vi "REF add remove phase element.vi"(1 "NewVal in":T1 {"REF phi (°)" format="%#_3g"}) -> (0 "NewVal out":T1 {"REF phi (°)" format="%#_3g"})   [LabVIEW 2016, in "Instrument.Lockin.lvclass"]
uses:
  Instrument.Lockin.lvclass
  LockinDAQ/Typedefs/REF-cluster.ctl
  LockinDAQ/Typedefs/REF_f-array.ctl
  LockinDAQ/Typedefs/REF_phi-array.ctl
  LockinDAQ/LockinDAQ.lvclass
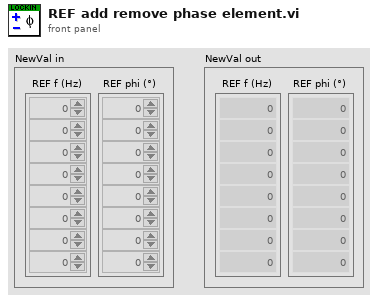
[diagram p1: front panel]
types:
  T1 = typedef "LockinDAQ.lvclass/REF-cluster.ctl" = cluster{"REF f (Hz)":T2, "REF phi (°)":T3}
  T2 = typedef "LockinDAQ.lvclass/REF_f-array.ctl" = dbl[]
  T3 = typedef "LockinDAQ.lvclass/REF_phi-array.ctl" = dbl[]
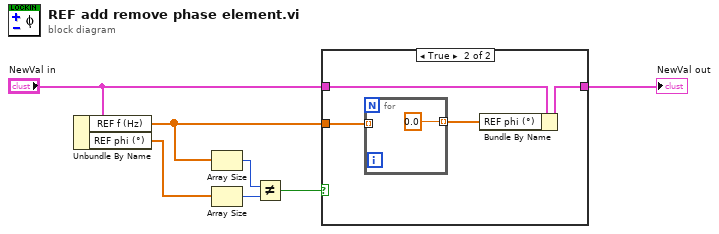
[diagram p0: block diagram]
diagram:
  n1 = Unbundle By Name("NewVal in") -> ("REF f (Hz)"=w6:T2, "REF phi (°)"=w5:T3)
  n2 = Array Size(array=w6) -> (size(s)=w4:i32)
  n3 = Array Size(array=w5) -> (size(s)=w7:i32)
  n4 = Not Equal?(x=w4, y=w7) -> (x != y?=w3:bool)
  n5 = case shown="True" w3 {
    tunnel: w6 -> [_ w12]
    tunnel: "NewVal in" -> [w8 w10]
    tunnel: [w8 w9] -> w1
    frame False {
    }
    frame True {
      n6 = for {
        tunnel: w12 -> [_] mode=indexing
        tunnel: [0.0] -> w11 mode=indexing
      }
      n7 = Bundle By Name(cluster=w10, "REF phi (°)"=w11) -> (w9:T1)
    }
  }
  "NewVal out" <- w1
